vi "GUI_Bella_1BL.vi"() -> ()   [LabVIEW 2020]
uses:
  Shared/GUI_Template/GUI_master/tcp_new_data_event.ctl
  Shared/GUI_Template/GUI_master/tcp new data cluster.ctl
  <vilib>/vision/Image Controls.llb/IMAQ Image.ctl
  <vilib>/ErrorRing/Error Ring.xnode
panel:
  in  "TargetSize.Y::6":dbl=430.0 caption="Size Y" min=2.0 max=3000.0
  in  "TargetSize.Y::7":dbl=20.0 caption="Size Y" min=2.0 max=3000.0
  in  "TargetSize.Y::8":dbl=20.0 caption="Size Y" min=2.0 max=3000.0
  in  "Thickness 8":u8=3
  in  "Thickness 7":u8=3
  in  "Thickness 6":u8=3
  in  "Thickness 5":u8=3
  in  "TargetSize.Y::5":dbl=150.0 caption="Size Y" min=2.0 max=3000.0
  in  "Thickness 4":u8=3
  in  "Thickness 3":u8=3
  in  "Thickness2":u8=3
  in  "TargetSize.Y::2":dbl=210.0 caption="Size Y" min=2.0 max=3000.0
  in  "TargetSize.Y::4":dbl=150.0 caption="Size Y" min=2.0 max=3000.0
  in  "Thickness":u8=3
  in  "TargetSize.Y::1":dbl=400.0 caption="Size Y" min=2.0 max=3000.0
  in  "TargetSize.Y::3":dbl=125.0 caption="Size Y" min=2.0 max=3000.0
  in  "Color":u32(colorbox)=16711680
  in  "Color 2":u32(colorbox)=16711680 caption="Color"
  in  "Color 3":u32(colorbox)=16711680 caption="Color"
  in  "Color 4":u32(colorbox)=16711680 caption="Color"
  in  "Color 5":u32(colorbox)=16711680 caption="Color"
  in  "Color 6":u32(colorbox)=16711680 caption="Color"
  in  "Color 7":u32(colorbox)=16711680 caption="Color"
  in  "Color 8":u32(colorbox)=16713728 caption="Color"
  out "Display8":T1(plugin-control) caption="M1 Cam"
  in  "Target.X::8":dbl=0.001 caption="X" min=0.0 max=2000.0
  in  "Target.Y::8":dbl=0.001 caption="Y" min=0.0 max=2000.0
  in  "TargetSize.X::8":dbl=20.0 caption="Size X" min=2.0 max=3000.0
  out "Display7":T1(plugin-control) caption="M1 Cam"
  in  "Target.X::7":dbl=0.001 caption="X" min=0.0 max=2000.0
  in  "Target.Y::7":dbl=0.001 caption="Y" min=0.0 max=2000.0
  in  "TargetSize.X::7":dbl=20.0 caption="Size X" min=2.0 max=3000.0
  out "Display6":T1(plugin-control) caption="M1 Cam"
  in  "Target.X::6":dbl=0.001 caption="X" min=0.0 max=2000.0
  in  "Target.Y::6":dbl=0.001 caption="Y" min=0.0 max=2000.0
  in  "TargetSize.X::6":dbl=430.0 caption="Size X" min=2.0 max=3000.0
  out "error out":errorcluster
  in  "GUIdevice 7":string="CAM-1BL-M5" caption="CAMERA 7"
  in  "GUIdevice 6":string="CAM-1BL-M2Near" caption="CAMERA 6"
  in  "GUIdevice 8":string="CAM-1BL-Ghost" caption="CAMERA 8"
  out "image::7":T1(plugin-control) caption="M1 Cam"
  out "image::8":T1(plugin-control) caption="M1 Cam"
  in  "centroidx::6":dbl=0.001 caption="X" min=0.0 max=0.0
  in  "centroidy::7":dbl=0.001 caption="Y" min=0.0 max=0.0
  in  "centroidx::7":dbl=0.001 caption="X" min=0.0 max=0.0
  in  "exposure::7":dbl=0.001 caption="Exposure" min=3.8e-05 max=1.0 format="%_4p"
  in  "trigger::7":bool caption="Blank Button"
  in  "centroidy::6":dbl=0.001 caption="Y" min=0.0 max=0.0
  in  "exposure::8":dbl=0.001 caption="Exposure" min=3.8e-05 max=1.0 format="%_4p"
  in  "trigger::8":bool caption="Blank Button"
  in  "centroidy::8":dbl=0.001 caption="Y" min=0.0 max=0.0
  in  "centroidx::8":dbl=0.001 caption="X" min=0.0 max=0.0
  in  "exposure::6":dbl=0.001 caption="Exposure" min=3.8e-05 max=1.0 format="%_4p"
  in  "trigger::6":bool caption="Blank Button"
  in  "image::6":T1(plugin-control) caption="M1 Cam"
  in  "roi::6":bool caption="Blank Button"
  in  "roi::7":bool caption="Blank Button"
  in  "roi::8":bool caption="Blank Button"
  out "Display5":T1(plugin-control) caption="M1 Cam"
  in  "Target.X::5":dbl=0.001 caption="X" min=0.0 max=2000.0
  in  "Target.Y::5":dbl=0.001 caption="Y" min=0.0 max=2000.0
  in  "TargetSize.X::5":dbl=150.0 caption="Size X" min=2.0 max=3000.0
  out "Display4":T1(plugin-control) caption="M1 Cam"
  in  "Target.X::4":dbl=0.001 caption="X" min=0.0 max=2000.0
  in  "Target.Y::4":dbl=0.001 caption="Y" min=0.0 max=2000.0
  in  "TargetSize.X::4":dbl=200.0 caption="Size" min=2.0 max=3000.0
  out "Display3":T1(plugin-control) caption="M1 Cam"
  in  "Target.X::3":dbl=0.001 caption="X" min=0.0 max=2000.0
  in  "Target.Y::3":dbl=0.001 caption="Y" min=0.0 max=2000.0
  in  "TargetSize.X::3":dbl=170.0 caption="Size X" min=2.0 max=3000.0
  in  "Target.X::2":dbl=0.001 caption="X" min=0.0 max=2000.0
  in  "Target.Y::2":dbl=0.001 caption="Y" min=0.0 max=2000.0
  in  "TargetSize.X::2":dbl=210.0 caption="Size X" min=2.0 max=3000.0
  out "Display2":T1(plugin-control) caption="M1 Cam"
  in  "roi::5":bool caption="Blank Button"
  in  "centroidx::5":dbl=0.001 caption="X" min=0.0 max=0.0
  in  "centroidy::5":dbl=0.001 caption="Y" min=0.0 max=0.0
  in  "trigger::5":bool caption="Blank Button"
  in  "exposure::5":dbl=0.001 caption="Exposure" min=3.8e-05 max=1.0 format="%_4p"
  in  "GUIdevice 5":string="CAM-1BL-M1" caption="CAMERA 5"
  in  "roi::4":bool caption="Blank Button"
  in  "centroidx::4":dbl=0.001 caption="X" min=0.0 max=0.0
  in  "centroidy::4":dbl=0.001 caption="Y" min=0.0 max=0.0
  in  "trigger::4":bool caption="Blank Button"
  in  "exposure::4":dbl=0.001 caption="Exposure" min=3.8e-05 max=1.0 format="%_4p"
  in  "GUIdevice 4":string="CAM-LT-Comp-IN" caption="CAMERA 4"
  in  "roi::3":bool caption="Blank Button"
  in  "centroidx::3":dbl=0.001 caption="X" min=0.0 max=0.0
  in  "centroidy::3":dbl=0.001 caption="Y" min=0.0 max=0.0
  in  "trigger::3":bool caption="Blank Button"
  in  "exposure::3":dbl=0.001 caption="Exposure" min=3.8e-05 max=1.0 format="%_4p"
  in  "GUIdevice 3":string="CAM-1BL-ShotControl" caption="CAMERA 3"
  in  "roi::1":bool caption="Blank Button"
  in  "TargetSize.X::1":dbl=410.0 caption="Size X" min=2.0 max=3000.0
  in  "Target.X::1":dbl=0.001 caption="X" min=0.0 max=2000.0
  in  "Target.Y::1":dbl=0.001 caption="Y" min=0.0 max=2000.0
  in  "centroidx::1":dbl=0.001 caption="X" min=0.0 max=0.0
  in  "centroidy::1":dbl=0.001 caption="Y" min=0.0 max=0.0
  in  "trigger::1":bool caption="Blank Button"
  in  "exposure::1":dbl=0.001 caption="Exposure" min=3.8e-05 max=1.0 format="%_4p"
  in  "GUIdevice 1":string="CAM-LT-Amp3Leak" caption="CAMERA 1"
  out "Display1":T1(plugin-control) caption="M1 Cam"
  in  "roi::2":bool caption="Blank Button"
  in  "centroidx::2":dbl=0.001 caption="X" min=0.0 max=0.0
  in  "centroidy::2":dbl=0.001 caption="Y" min=0.0 max=0.0
  in  "trigger::2":bool caption="Blank Button"
  in  "exposure::2":dbl=0.001 caption="Exposure" min=3.8e-05 max=1.0 format="%_4p"
  in  "GUIdevice 2":string="CAM-1BL-DM" caption="CAMERA 2"
  out "image::5":T1(plugin-control) caption="M1 Cam"
  out "image::4":T1(plugin-control) caption="M1 Cam"
  in  "image::3":T1(plugin-control) caption="M1 Cam"
  out "image::2":T1(plugin-control) caption="M1 Cam"
  out "image::1":T1(plugin-control) caption="M1 Cam"
  out "tcp data event":T2
  in  "stop":bool
  out "error IO 2":errorcluster
  # "1BL GUI - 1"
  # "Target"
  # "Centroid"
  # "Target"
  # "Centroid"
  # "Target"
  # "Target"
  # "Centroid"
  # "Centroid"
  # "Target"
  # "Target"
  # "Target"
  # "Centroid"
  # "Centroid"
  # "Centroid"
  # "Target"
  # "Centroid"
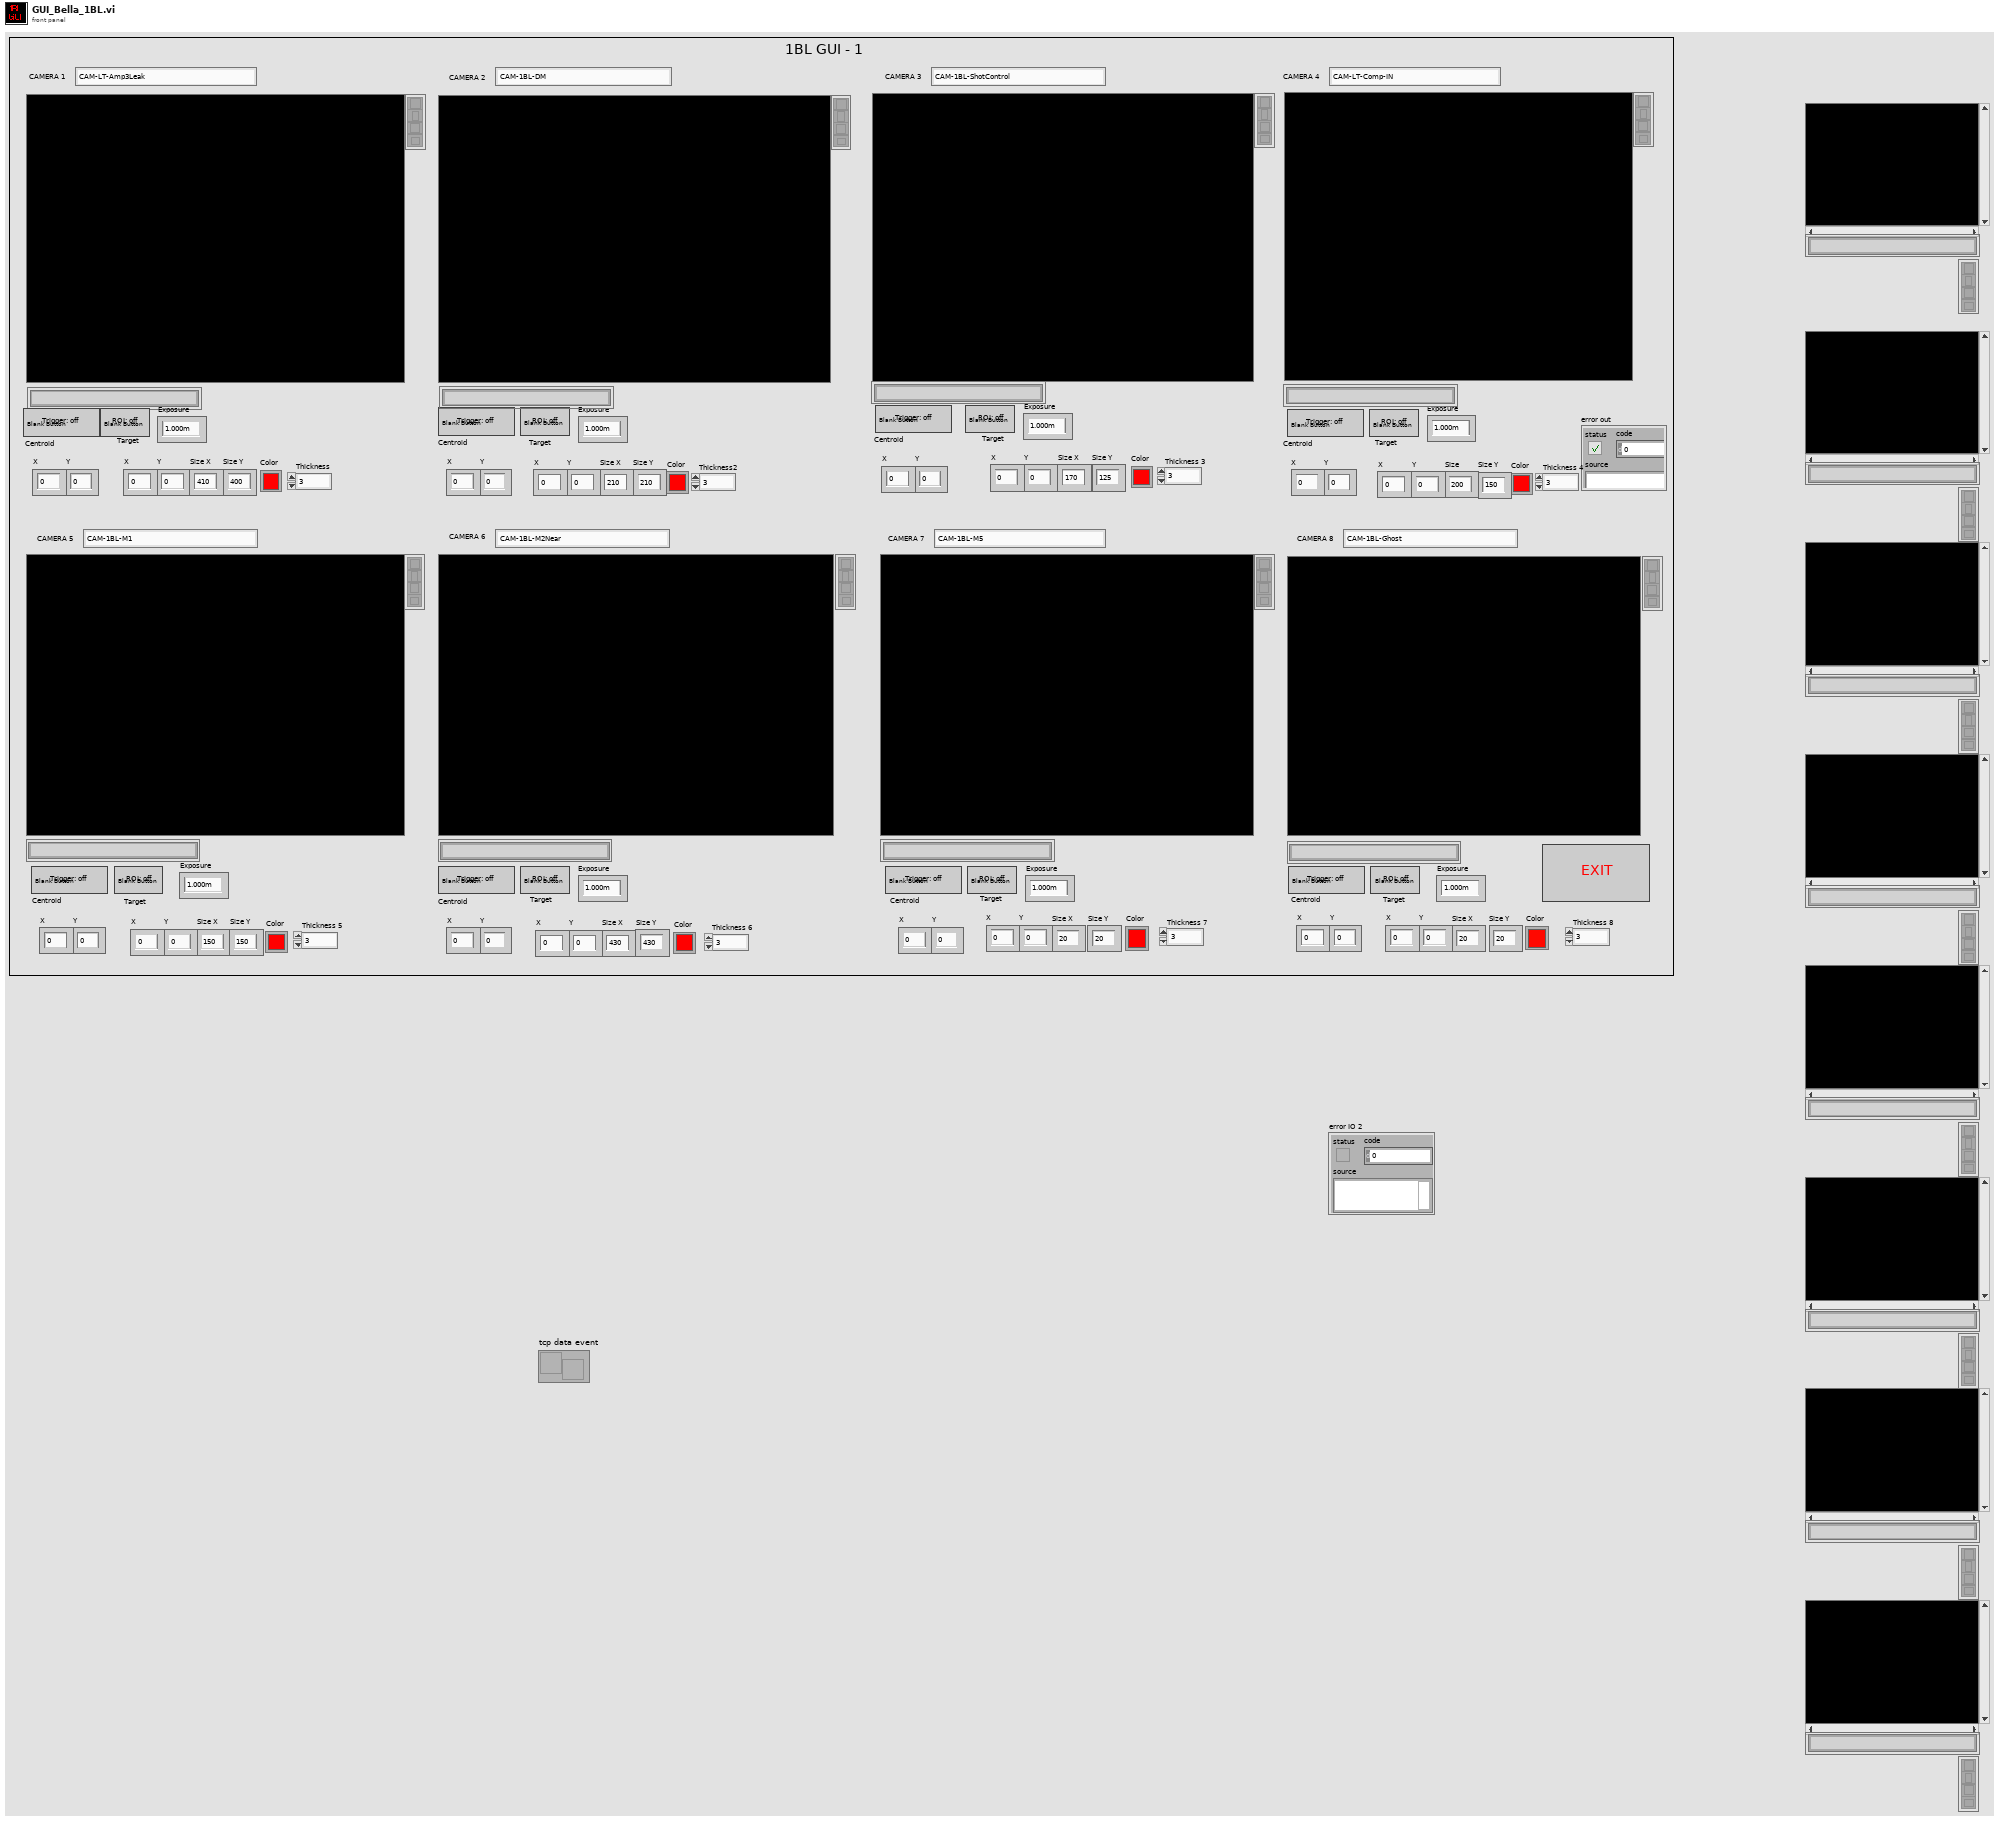
[diagram p1: front panel]
types:
  T1 = typedef "IMAQ Image.ctl" = refnum<image>
  T2 = typedef "tcp_new_data_event.ctl" = refnum<user-event>
  T3 = cluster{"Image1":T1, "Image2":T1, "Image3":T1, "Image4":T1, "Image5":T1, "Image6":T1, "Image7":T1, "Image8":T1}
  T4 = cluster{"Last update Cam1":u32, "Last update Cam2":u32, "Last update Cam3":u32, "Last update Cam4":u32, "Last update Cam5":u32, "Last update Cam6":u32, "Last update Cam7":u32, "Last update Cam8":u32}
  T5 = typedef "Image Type" = u32
  T6 = typedef "tcp new data cluster.ctl" = cluster{"EventEnum":enum16{"new data", "connection status update"}, "Device name":string}
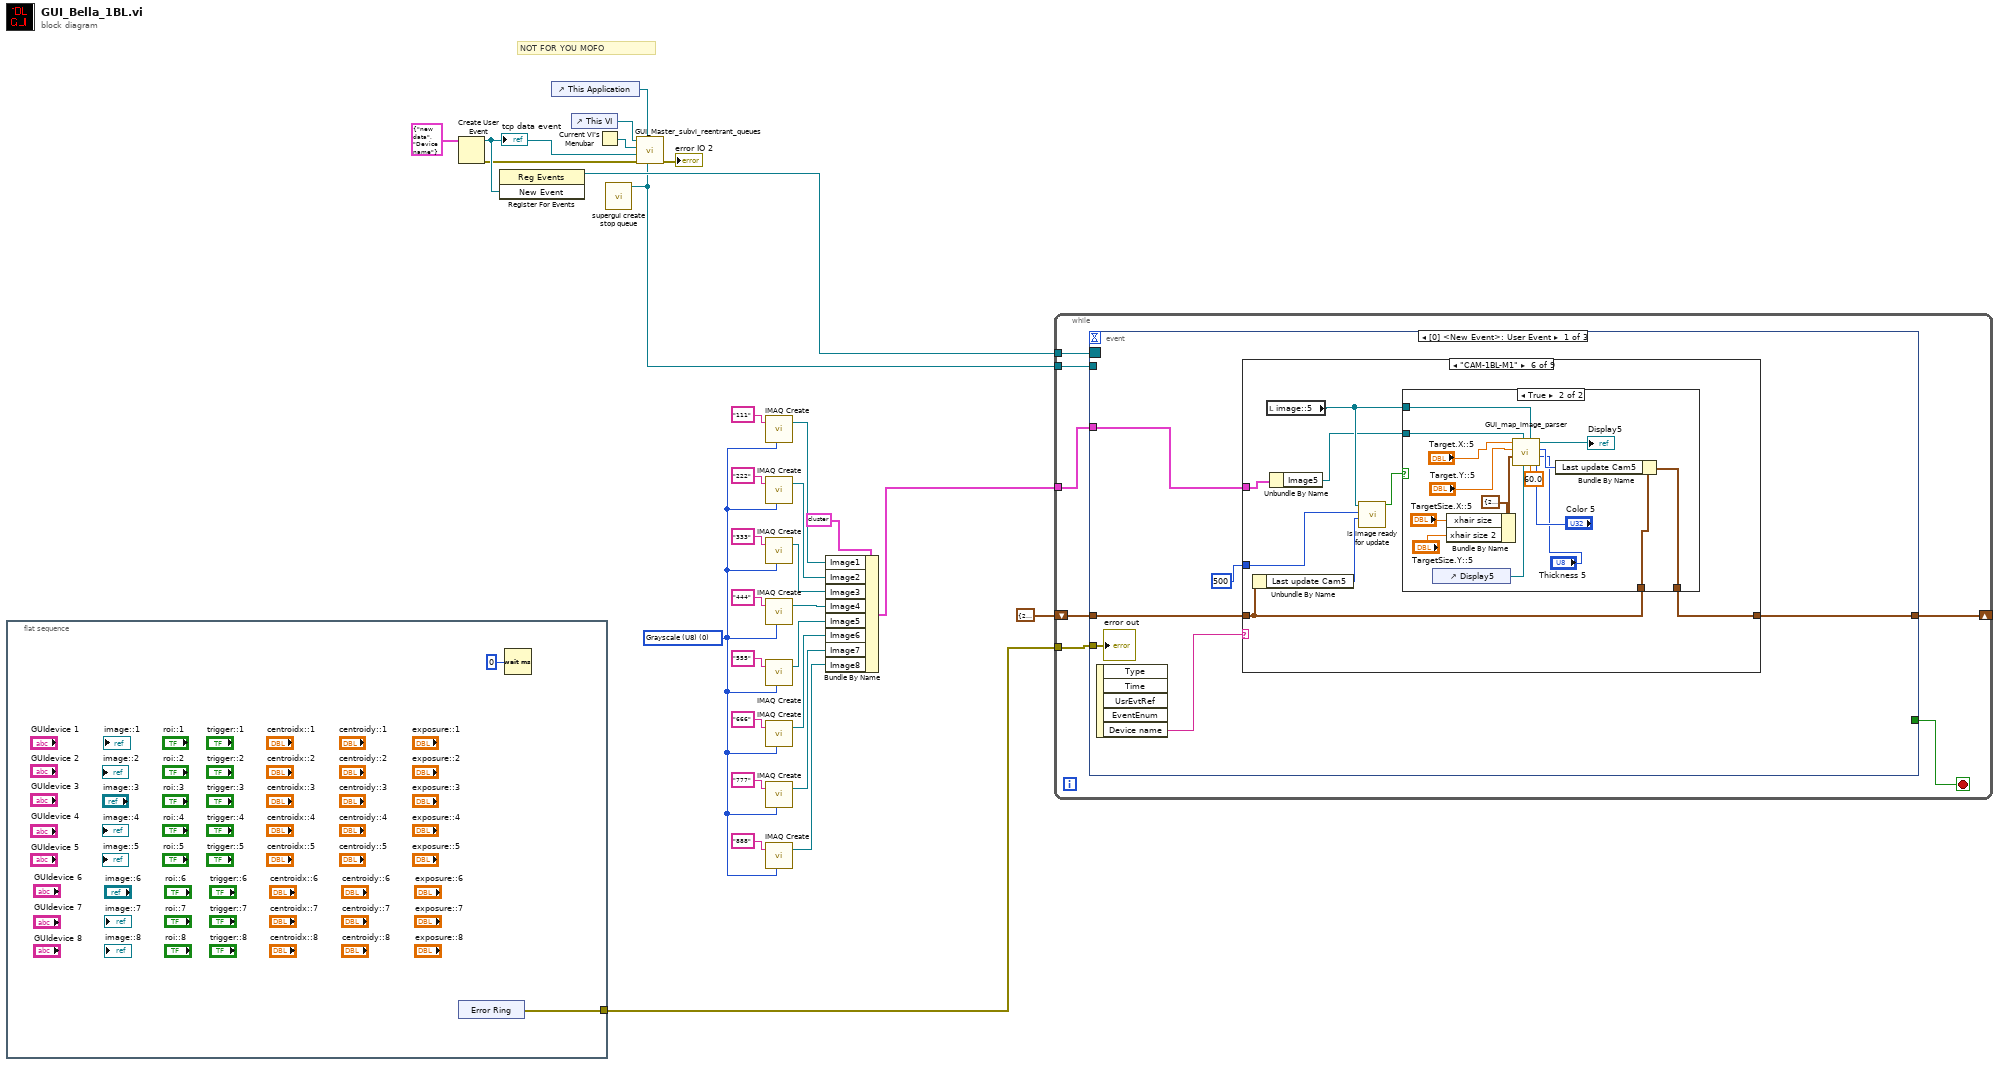
[diagram p0: block diagram]
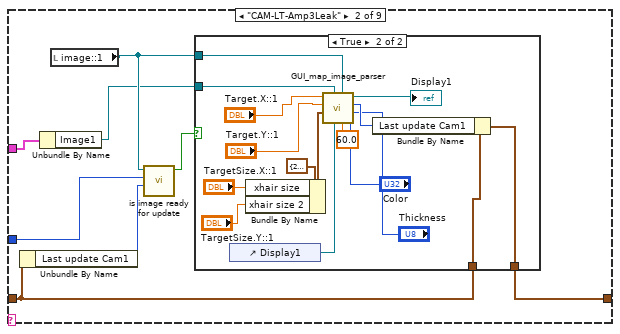
[diagram p3: hidden frame]
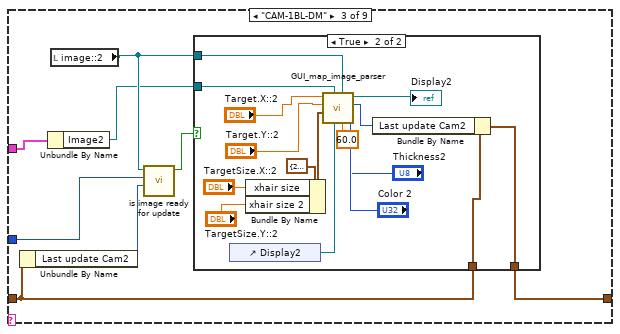
[diagram p5: hidden frame]
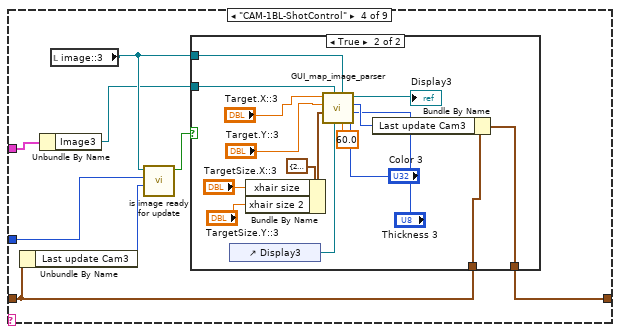
[diagram p7: hidden frame]
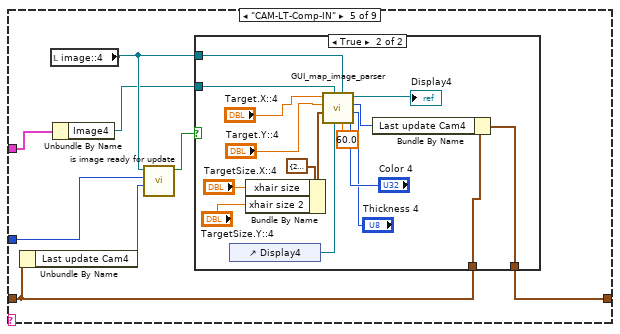
[diagram p9: hidden frame]
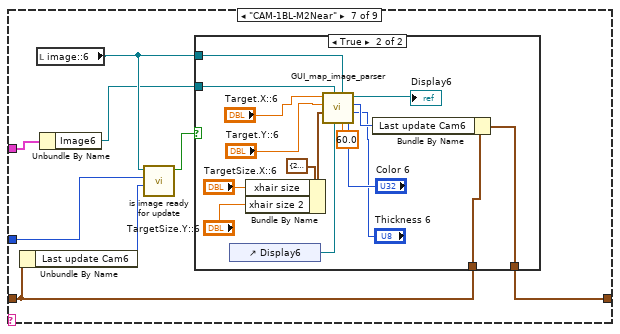
[diagram p12: hidden frame]
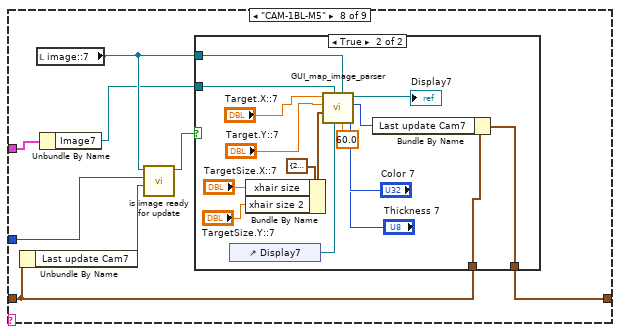
[diagram p14: hidden frame]
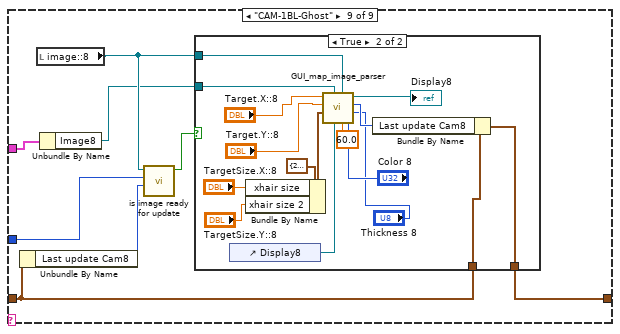
[diagram p16: hidden frame]
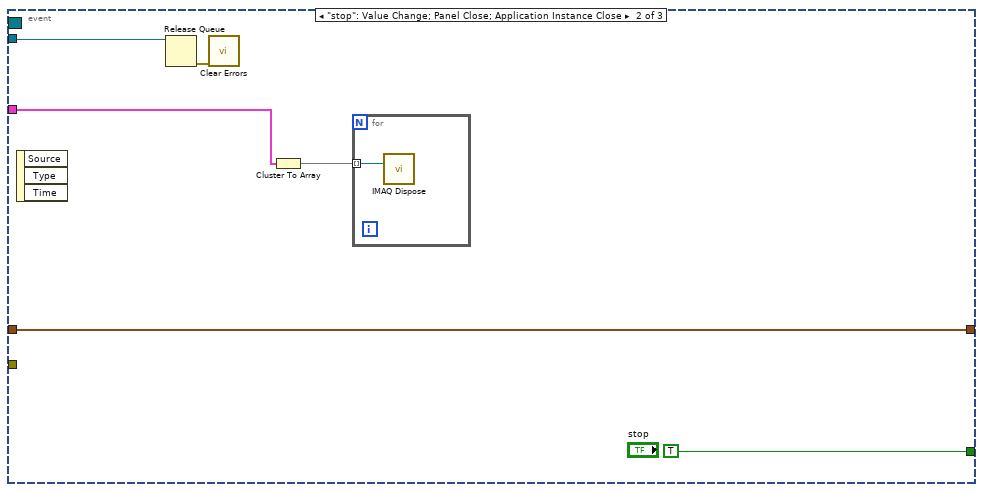
[diagram p18: hidden frame]
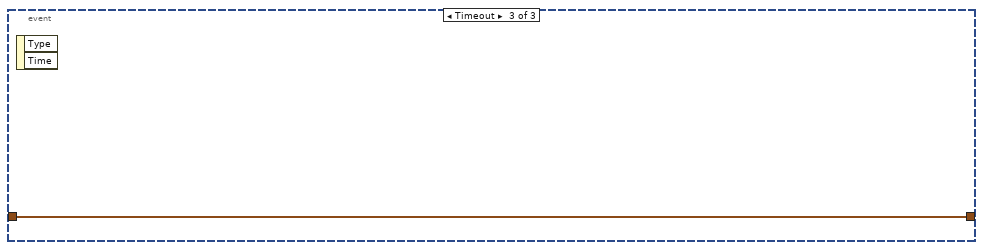
[diagram p19: hidden frame]
diagram:
  w12 = T5 0 items=["Grayscale (U8)", "Grayscale (I16)", "Grayscale (SGL)", "Complex (CSG)", "RGB (U32)", "HSL (U32)", "RGB (U64)", "Grayscale (U16)"] ("Image Type")
  # "NOT FOR YOU MOFO"
  n1 = flat-sequence {
    tunnel: [w32] -> w1
    frame #0 {
      n2 = xnode "Error Ring"() -> ("error out"=w32:errorcluster)
      n3 = Wait (ms)(milliseconds to wait=u32 0) -> ()  [unwired: 1 out]
    }
  }
  n4 = Create User Event(user event datatype=T6 {"EventEnum"=enum."new data", "Device name"="Device name"} ("New Event")) -> (user event=w29:refnum<user-event>, error out=w28:errorcluster)  [unwired: 1 in]
  "tcp data event" <- w29
  n5 = register-events(w29) -> (reference out=w24:refnum<event-registration>)  [unwired: 2 in, 1 out]
  n6 = control-ref of="This Application"() -> (w30:refnum<vi>)
  n7 = control-ref of="This VI"() -> (w25:refnum<vi>)
  n8 = Current VI's Menubar() -> (w26:refnum<k9>)
  n9 = call "supergui create stop queue.vi"() -> ("STOP Queue out"=w16:refnum<queue>)  [unwired: 11 in]
  n10 = call "GUI_Master_subvi_reentrant_queues.vi"("STOP Queue in"=w16, "This Application"=w30, "error in (no error)"=w28, "tcp data event"=w29, "Caller menu reference"=w26, "Caller VI ref"=w25) -> ("error out"=→"error IO 2":errorcluster)  [unwired: 5 in]
  n11 = call "IMAQ Create"("Image Name"="111", "Image Type"=w12) -> ("New Image"=w11:T1)  [unwired: 3 in, 1 out]
  n12 = call "IMAQ Create"("Image Name"="222", "Image Type"=w12) -> ("New Image"=w10:T1)  [unwired: 3 in, 1 out]
  n13 = call "IMAQ Create"("Image Name"="333", "Image Type"=w12) -> ("New Image"=w9:T1)  [unwired: 3 in, 1 out]
  n14 = call "IMAQ Create"("Image Name"="444", "Image Type"=w12) -> ("New Image"=w8:T1)  [unwired: 3 in, 1 out]
  n15 = call "IMAQ Create"("Image Name"="555", "Image Type"=w12) -> ("New Image"=w7:T1)  [unwired: 3 in, 1 out]
  n16 = call "IMAQ Create"("Image Name"="666", "Image Type"=w12) -> ("New Image"=w6:T1)  [unwired: 3 in, 1 out]
  n17 = call "IMAQ Create"("Image Name"="777", "Image Type"=w12) -> ("New Image"=w5:T1)  [unwired: 3 in, 1 out]
  n18 = call "IMAQ Create"("Image Name"="888", "Image Type"=w12) -> ("New Image"=w4:T1)  [unwired: 3 in, 1 out]
  n19 = Bundle By Name(cluster=T3 {"Image1"=refnum, "Image2"=refnum, "Image3"=refnum, "Image4"=refnum, "Image5"=refnum, "Image6"=refnum, "Image7"=refnum, "Image8"=refnum}, "Image1"=w11, "Image2"=w10, "Image3"=w9, "Image4"=w8, "Image5"=w7, "Image6"=w6, "Image7"=w5, "Image8"=w4) -> (w2:T3)
  n20 = while {
    tunnel: w24 -> [w39]
    shift-right: [w37] -> _
    shift-left: T4 {"Last update Cam1"=200, "Last update Cam2"=200, "Last update Cam3"=200, "Last update Cam4"=200, "Last update Cam5"=200, "Last update Cam6"=200, "Last update Cam7"=200, "Last update Cam8"=200} -> [w38]
    tunnel: w16 -> [w36]
    tunnel: w2 -> [w35]
    tunnel: w1 -> [w34]
    stop <- w40 stop-if-true
    n21 = event shown="[0] <New Event>: User Event" {
      selector: w39 -> [_ _ _]
      dyn-events: _ -> [_ _ _]
      timeout: _ -> [_ _ _]
      tunnel: [_ TRUE ("stop") _] -> w40
      tunnel: w38 -> [w45 w252 w255]
      tunnel: [w43 w252 w255] -> w37
      tunnel: w36 -> [_ w251 _]
      tunnel: w35 -> [w42 w249 _]
      tunnel: w34 -> [w41 _ _]
      event User Event {
        n22 = event-data() -> ("Device name"=w46:string)  [unwired: 1 in, 4 out]
        n23 = case shown="\"CAM-1BL-M1\"" w46 {
          tunnel: w45 -> [w47 w55 w80 w105 w130 w155 w180 w205 w230]
          tunnel: u32 500 ("x-y") -> [_ w53 w78 w103 w128 w153 w178 w203 w228]
          tunnel: [w47 w54 w79 w104 w129 w154 w179 w204 w229] -> w43
          tunnel: w42 -> [_ w49 w74 w99 w124 w149 w174 w199 w224]
          frame Default {
          }
          frame "CAM-LT-Amp3Leak" {
            n24 = Unbundle By Name(w55) -> ("Last update Cam1"=w52:u32)
            n25 = Unbundle By Name(w49) -> ("Image1"=w48:T1)
            n26 = local read "image::1"() -> (w50:T1)
            n27 = call "is image ready for update.vi"("Last update"=w52, "min time between updates"=w53, "image ref in"=w50) -> ("update image"=w51:bool)  [unwired: 8 in]
            n28 = case shown="True" w51 {
              tunnel: w55 -> [w56 w72]
              tunnel: [w56 w71] -> w54
              tunnel: w50 -> [_ w70]
              tunnel: w48 -> [_ w60]
              frame False {
              }
              frame True {
                n29 = control-ref of="Display1"() -> (w66:refnum<vi>)
                n30 = Bundle By Name(cluster=cluster{"xhair size":dbl, "xhair size 2":dbl} {"xhair size"=20.0, "xhair size 2"=20.0} ("size"), "xhair size"="TargetSize.X::1", "xhair size 2"="TargetSize.Y::1") -> (w61:cluster{"xhair size":dbl, "xhair size 2":dbl})
                n31 = call "GUI_map_image_parser.vi"("color"="Color", "Thickness"="Thickness", "zoom#"=60.0, "Image Src"=w70, "Ctl Refnum"=w66, "Image Dst"=w60, "size"=w61, "target y"="Target.Y::1", "target x"="Target.X::1") -> ("ms timer out"=w65:u32, "Img out"=→"Display1":T1)  [unwired: 1 in]
                n32 = Bundle By Name(cluster=w72, "Last update Cam1"=w65) -> (w71:T4)
              }
            }
          }
          frame "CAM-1BL-DM" {
            n33 = Unbundle By Name(w80) -> ("Last update Cam2"=w77:u32)
            n34 = Unbundle By Name(w74) -> ("Image2"=w73:T1)
            n35 = local read "image::2"() -> (w75:T1)
            n36 = call "is image ready for update.vi"("Last update"=w77, "min time between updates"=w78, "image ref in"=w75) -> ("update image"=w76:bool)  [unwired: 8 in]
            n37 = case shown="True" w76 {
              tunnel: w80 -> [w81 w97]
              tunnel: [w81 w96] -> w79
              tunnel: w75 -> [_ w95]
              tunnel: w73 -> [_ w85]
              frame False {
              }
              frame True {
                n38 = control-ref of="Display2"() -> (w91:refnum<vi>)
                n39 = Bundle By Name(cluster=cluster{"xhair size":dbl, "xhair size 2":dbl} {"xhair size"=20.0, "xhair size 2"=20.0} ("size"), "xhair size"="TargetSize.X::2", "xhair size 2"="TargetSize.Y::2") -> (w86:cluster{"xhair size":dbl, "xhair size 2":dbl})
                n40 = call "GUI_map_image_parser.vi"("color"="Color 2", "Thickness"="Thickness2", "zoom#"=60.0, "Image Src"=w95, "Ctl Refnum"=w91, "Image Dst"=w85, "size"=w86, "target y"="Target.Y::2", "target x"="Target.X::2") -> ("ms timer out"=w90:u32, "Img out"=→"Display2":T1)  [unwired: 1 in]
                n41 = Bundle By Name(cluster=w97, "Last update Cam2"=w90) -> (w96:T4)
              }
            }
          }
          frame "CAM-1BL-ShotControl" {
            n42 = Unbundle By Name(w105) -> ("Last update Cam3"=w102:u32)
            n43 = Unbundle By Name(w99) -> ("Image3"=w98:T1)
            n44 = local read "image::3"() -> (w100:T1)
            n45 = call "is image ready for update.vi"("Last update"=w102, "min time between updates"=w103, "image ref in"=w100) -> ("update image"=w101:bool)  [unwired: 8 in]
            n46 = case shown="True" w101 {
              tunnel: w105 -> [w106 w122]
              tunnel: [w106 w121] -> w104
              tunnel: w100 -> [_ w120]
              tunnel: w98 -> [_ w110]
              frame False {
              }
              frame True {
                n47 = control-ref of="Display3"() -> (w116:refnum<vi>)
                n48 = Bundle By Name(cluster=cluster{"xhair size":dbl, "xhair size 2":dbl} {"xhair size"=20.0, "xhair size 2"=20.0} ("size"), "xhair size"="TargetSize.X::3", "xhair size 2"="TargetSize.Y::3") -> (w111:cluster{"xhair size":dbl, "xhair size 2":dbl})
                n49 = call "GUI_map_image_parser.vi"("color"="Color 3", "Thickness"="Thickness 3", "zoom#"=60.0, "Image Src"=w120, "Ctl Refnum"=w116, "Image Dst"=w110, "size"=w111, "target y"="Target.Y::3", "target x"="Target.X::3") -> ("ms timer out"=w115:u32, "Img out"=→"Display3":T1)  [unwired: 1 in]
                n50 = Bundle By Name(cluster=w122, "Last update Cam3"=w115) -> (w121:T4)
              }
            }
          }
          frame "CAM-LT-Comp-IN" {
            n51 = Unbundle By Name(w130) -> ("Last update Cam4"=w127:u32)
            n52 = local read "image::4"() -> (w125:T1)
            n53 = Unbundle By Name(w124) -> ("Image4"=w123:T1)
            n54 = call "is image ready for update.vi"("Last update"=w127, "min time between updates"=w128, "image ref in"=w125) -> ("update image"=w126:bool)  [unwired: 8 in]
            n55 = case shown="True" w126 {
              tunnel: w130 -> [w131 w147]
              tunnel: [w131 w146] -> w129
              tunnel: w125 -> [_ w145]
              tunnel: w123 -> [_ w135]
              frame False {
              }
              frame True {
                n56 = control-ref of="Display4"() -> (w141:refnum<vi>)
                n57 = Bundle By Name(cluster=cluster{"xhair size":dbl, "xhair size 2":dbl} {"xhair size"=20.0, "xhair size 2"=20.0} ("size"), "xhair size"="TargetSize.X::4", "xhair size 2"="TargetSize.Y::4") -> (w136:cluster{"xhair size":dbl, "xhair size 2":dbl})
                n58 = call "GUI_map_image_parser.vi"("color"="Color 4", "Thickness"="Thickness 4", "zoom#"=60.0, "Image Src"=w145, "Ctl Refnum"=w141, "Image Dst"=w135, "size"=w136, "target y"="Target.Y::4", "target x"="Target.X::4") -> ("ms timer out"=w140:u32, "Img out"=→"Display4":T1)  [unwired: 1 in]
                n59 = Bundle By Name(cluster=w147, "Last update Cam4"=w140) -> (w146:T4)
              }
            }
          }
          frame "CAM-1BL-M1" {
            n60 = Unbundle By Name(w155) -> ("Last update Cam5"=w152:u32)
            n61 = local read "image::5"() -> (w150:T1)
            n62 = Unbundle By Name(w149) -> ("Image5"=w148:T1)
            n63 = call "is image ready for update.vi"("Last update"=w152, "min time between updates"=w153, "image ref in"=w150) -> ("update image"=w151:bool)  [unwired: 8 in]
            n64 = case shown="True" w151 {
              tunnel: w155 -> [w156 w172]
              tunnel: [w156 w171] -> w154
              tunnel: w150 -> [_ w170]
              tunnel: w148 -> [_ w161]
              frame False {
              }
              frame True {
                n65 = control-ref of="Display5"() -> (w166:refnum<vi>)
                n66 = Bundle By Name(cluster=cluster{"xhair size":dbl, "xhair size 2":dbl} {"xhair size"=20.0, "xhair size 2"=20.0} ("size"), "xhair size"="TargetSize.X::5", "xhair size 2"="TargetSize.Y::5") -> (w162:cluster{"xhair size":dbl, "xhair size 2":dbl})
                n67 = call "GUI_map_image_parser.vi"("color"="Color 5", "Thickness"="Thickness 5", "zoom#"=60.0, "Image Src"=w170, "Ctl Refnum"=w166, "Image Dst"=w161, "size"=w162, "target y"="Target.Y::5", "target x"="Target.X::5") -> ("ms timer out"=w165:u32, "Img out"=→"Display5":T1)  [unwired: 1 in]
                n68 = Bundle By Name(cluster=w172, "Last update Cam5"=w165) -> (w171:T4)
              }
            }
          }
          frame "CAM-1BL-M2Near" {
            n69 = Unbundle By Name(w180) -> ("Last update Cam6"=w177:u32)
            n70 = local read "image::6"() -> (w175:T1)
            n71 = Unbundle By Name(w174) -> ("Image6"=w173:T1)
            n72 = call "is image ready for update.vi"("Last update"=w177, "min time between updates"=w178, "image ref in"=w175) -> ("update image"=w176:bool)  [unwired: 8 in]
            n73 = case shown="True" w176 {
              tunnel: w180 -> [w181 w197]
              tunnel: [w181 w196] -> w179
              tunnel: w175 -> [_ w195]
              tunnel: w173 -> [_ w185]
              frame False {
              }
              frame True {
                n74 = control-ref of="Display6"() -> (w191:refnum<vi>)
                n75 = Bundle By Name(cluster=cluster{"xhair size":dbl, "xhair size 2":dbl} {"xhair size"=20.0, "xhair size 2"=20.0} ("size"), "xhair size"="TargetSize.X::6", "xhair size 2"="TargetSize.Y::6") -> (w186:cluster{"xhair size":dbl, "xhair size 2":dbl})
                n76 = call "GUI_map_image_parser.vi"("color"="Color 6", "Thickness"="Thickness 6", "zoom#"=60.0, "Image Src"=w195, "Ctl Refnum"=w191, "Image Dst"=w185, "size"=w186, "target y"="Target.Y::6", "target x"="Target.X::6") -> ("ms timer out"=w190:u32, "Img out"=→"Display6":T1)  [unwired: 1 in]
                n77 = Bundle By Name(cluster=w197, "Last update Cam6"=w190) -> (w196:T4)
              }
            }
          }
          frame "CAM-1BL-M5" {
            n78 = Unbundle By Name(w205) -> ("Last update Cam7"=w202:u32)
            n79 = local read "image::7"() -> (w200:T1)
            n80 = Unbundle By Name(w199) -> ("Image7"=w198:T1)
            n81 = call "is image ready for update.vi"("Last update"=w202, "min time between updates"=w203, "image ref in"=w200) -> ("update image"=w201:bool)  [unwired: 8 in]
            n82 = case shown="True" w201 {
              tunnel: w205 -> [w206 w222]
              tunnel: [w206 w221] -> w204
              tunnel: w200 -> [_ w220]
              tunnel: w198 -> [_ w210]
              frame False {
              }
              frame True {
                n83 = control-ref of="Display7"() -> (w216:refnum<vi>)
                n84 = Bundle By Name(cluster=cluster{"xhair size":dbl, "xhair size 2":dbl} {"xhair size"=20.0, "xhair size 2"=20.0} ("size"), "xhair size"="TargetSize.X::7", "xhair size 2"="TargetSize.Y::7") -> (w211:cluster{"xhair size":dbl, "xhair size 2":dbl})
                n85 = call "GUI_map_image_parser.vi"("color"="Color 7", "Thickness"="Thickness 7", "zoom#"=60.0, "Image Src"=w220, "Ctl Refnum"=w216, "Image Dst"=w210, "size"=w211, "target y"="Target.Y::7", "target x"="Target.X::7") -> ("ms timer out"=w215:u32, "Img out"=→"Display7":T1)  [unwired: 1 in]
                n86 = Bundle By Name(cluster=w222, "Last update Cam7"=w215) -> (w221:T4)
              }
            }
          }
          frame "CAM-1BL-Ghost" {
            n87 = Unbundle By Name(w230) -> ("Last update Cam8"=w227:u32)
            n88 = local read "image::8"() -> (w225:T1)
            n89 = Unbundle By Name(w224) -> ("Image8"=w223:T1)
            n90 = call "is image ready for update.vi"("Last update"=w227, "min time between updates"=w228, "image ref in"=w225) -> ("update image"=w226:bool)  [unwired: 8 in]
            n91 = case shown="True" w226 {
              tunnel: w230 -> [w231 w247]
              tunnel: [w231 w246] -> w229
              tunnel: w225 -> [_ w245]
              tunnel: w223 -> [_ w236]
              frame False {
              }
              frame True {
                n92 = control-ref of="Display8"() -> (w241:refnum<vi>)
                n93 = Bundle By Name(cluster=cluster{"xhair size":dbl, "xhair size 2":dbl} {"xhair size"=20.0, "xhair size 2"=20.0} ("size"), "xhair size"="TargetSize.X::8", "xhair size 2"="TargetSize.Y::8") -> (w237:cluster{"xhair size":dbl, "xhair size 2":dbl})
                n94 = call "GUI_map_image_parser.vi"("color"="Color 8", "Thickness"="Thickness 8", "zoom#"=60.0, "Image Src"=w245, "Ctl Refnum"=w241, "Image Dst"=w236, "size"=w237, "target y"="Target.Y::8", "target x"="Target.X::8") -> ("ms timer out"=w240:u32, "Img out"=→"Display8":T1)  [unwired: 1 in]
                n95 = Bundle By Name(cluster=w247, "Last update Cam8"=w240) -> (w246:T4)
              }
            }
          }
        }
        "error out" <- w41
      }
      event "stop": Value Change; Panel Close; Application Instance Close {
        n96 = event-data() -> ()  [unwired: 1 in, 3 out]
        n97 = Release Queue(queue=w251) -> (error out=w250:errorcluster)  [unwired: 2 in, 2 out]
        n98 = call <vilib>:"Clear Errors.vi"("error in (no error)"=w250) -> ()  [unwired: 5 in, 2 out]
        n99 = Cluster To Array(cluster=w249) -> (array=w248:T1[])
        n100 = for {
          tunnel: w248 -> [w254] mode=indexing
          n101 = call "IMAQ Dispose"("Image"=w254) -> ()  [unwired: 5 in, 1 out]
        }
      }
      event Timeout {
        n102 = event-data() -> ()  [unwired: 1 in, 2 out]
      }
    }
  }
